vi "Tosca-Configure Multirigs.vi"(2 "Parent VI":refnum<vi>) -> (8 "Canceled?":bool)   [LabVIEW 2020]
uses:
  epl-vi-lib/Utility VIs/Buttons/KCheckmarkBoolean 2.ctl
  epl-vi-lib/Utility VIs/Controls/KTable/KTable.xctl
panel:
  in  "KTable":u16(xcontrol)
  in  "Apply to all":T1
  in  "Edit defaults":bool
  in  "Cancel":bool
  in  "OK":bool
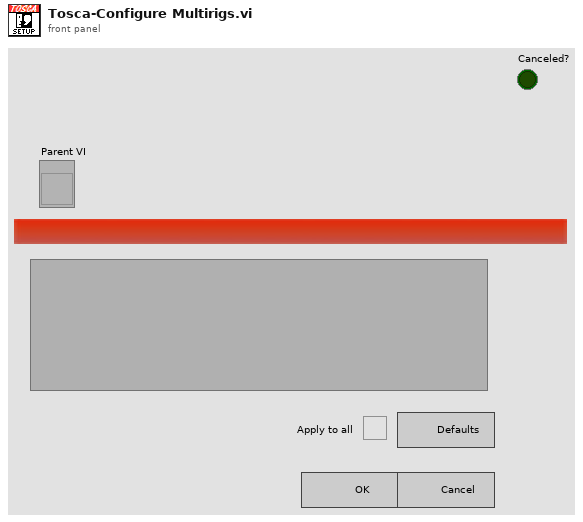
[diagram p1: front panel]
types:
  T1 = typedef "KCheckmarkBoolean 2.ctl" = bool
  T2 = cluster{"Name":string, "Audio":string, "Digital":string, "Video":string}[]
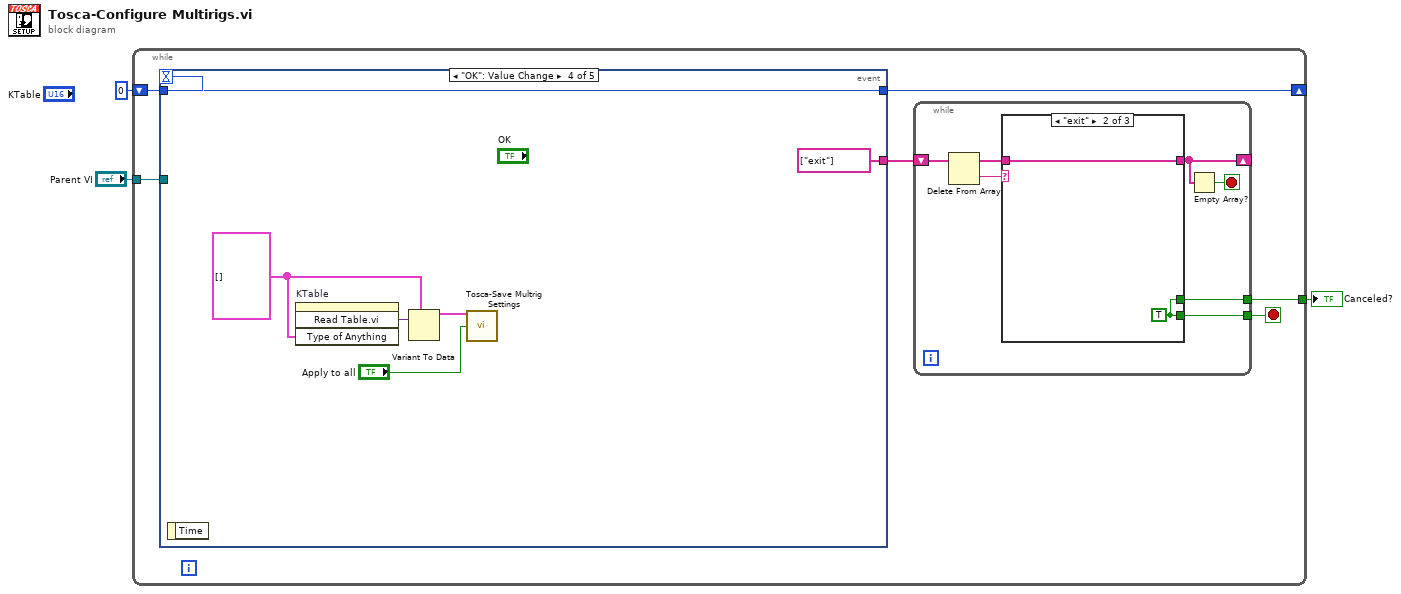
[diagram p0: block diagram]
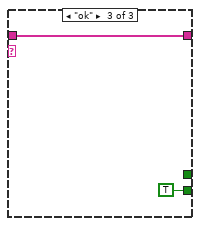
[diagram p3: hidden frame]
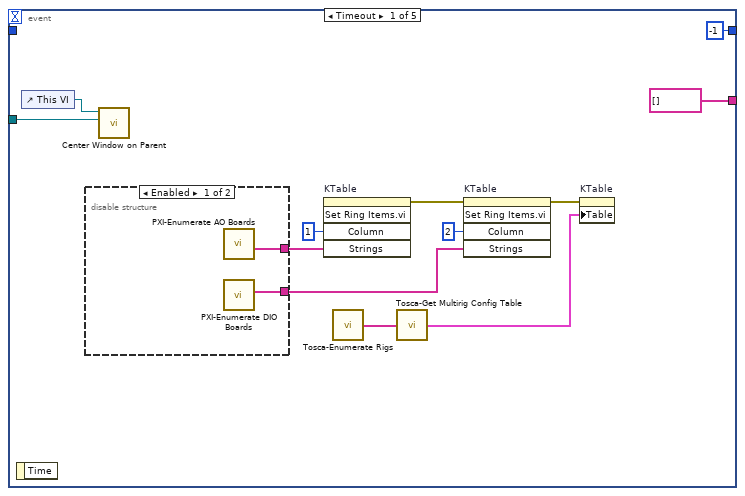
[diagram p4: hidden frame]
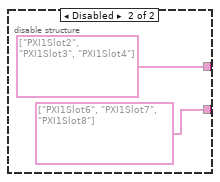
[diagram p5: hidden frame]
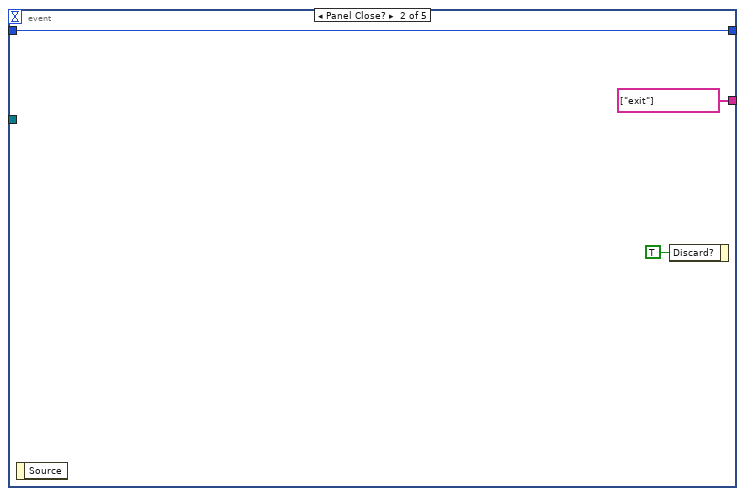
[diagram p6: hidden frame]
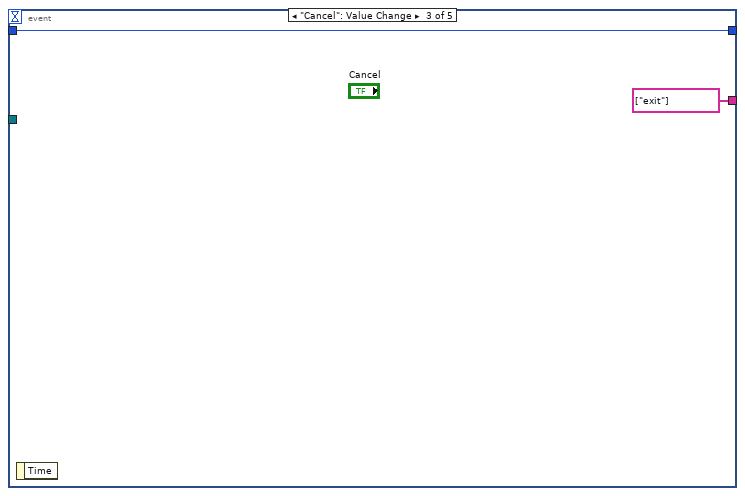
[diagram p7: hidden frame]
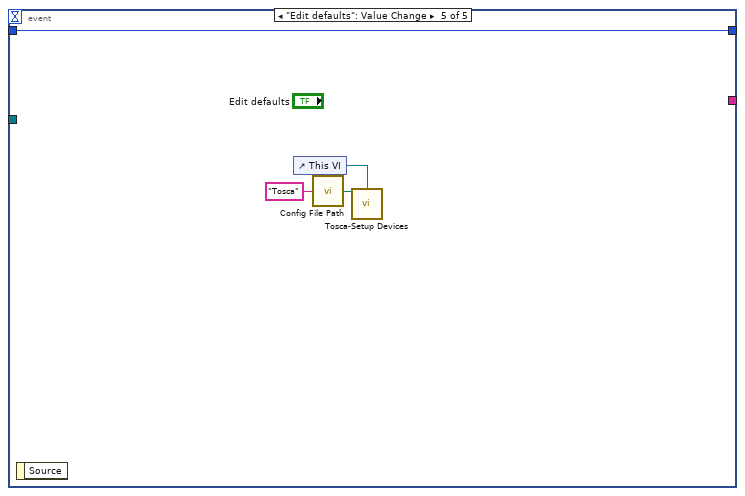
[diagram p8: hidden frame]
diagram:
  n1 = while {
    shift-right: [w9] -> _
    shift-left: 0 -> [w8]
    tunnel: [w5] -> w2
    tunnel: "Parent VI" -> [w4]
    stop <- w6 stop-if-true
    n2 = event shown="[3] \"OK\": Value Change" {
      selector: _ -> [_ _ _ _ _]
      dyn-events: _ -> [_ _ _ _ _]
      timeout: w8 -> [_ _ _ _ _]
      tunnel: [-1 w40 w42 w48 w52] -> w9
      tunnel: w8 -> [_ w40 w42 w48 w52]
      tunnel: [string[] [] string[] ["exit"] string[] ["exit"] string[] ["exit"] _] -> w7
      tunnel: w4 -> [w30 _ _ _ _]
      event Timeout {
        n3 = event-data() -> ()  [unwired: 1 in, 1 out]
        n4 = control-ref of="This VI"() -> (w31:refnum<vi>)
        n5 = disable-structure shown="Enabled" {
          disable-tunnel: [w34 string[] ["PXI1Slot2", "PXI1Slot3", "PXI1Slot4"]] -> w25
          disable-tunnel: [w35 string[] ["PXI1Slot6", "PXI1Slot7", "PXI1Slot8"]] -> w29
          frame Enabled {
            n6 = call "PXI-Enumerate AO Boards.vi"() -> ("24-bit devices"=w34:tag[])  [unwired: 9 in, 2 out]
            n7 = call "PXI-Enumerate DIO Boards.vi"() -> ("Devices"=w35:tag[])  [unwired: 10 in, 1 out]
          }
          frame Disabled {
          }
        }
        n8 = call "Center Window on Parent.vi"("Parent VI"=w30, "VI in"=w31) -> ()  [unwired: 8 in, 2 out]
        n9 = invoke on="KTable" class="KTable (strict)" method="Set Ring Items.vi"("Column"=1, "Strings"=w25) -> (error out=w27:errorcluster)  [unwired: 3 in, 4 out]
        n10 = call "Tosca-Enumerate Rigs.vi"() -> ("Rigs"=w24:string[])  [unwired: 15 in]
        n11 = call "Tosca-Get Multirig Config Table.vi"("Rigs"=w24) -> ("Table"=w22:T2)  [unwired: 14 in]
        n12 = invoke on="KTable" class="KTable (strict)" method="Set Ring Items.vi"(error in=w27, "Column"=2, "Strings"=w29) -> (error out=w23:errorcluster)  [unwired: 2 in, 4 out]
        n13 = property on="KTable" class="KTable (strict)"(error in=w23, "Table"=w22) -> ()  [unwired: 1 in, 2 out]
      }
      event Panel Close? {
        n14 = event-data() -> ()  [unwired: 1 in, 1 out]
        n15 = event-data("Discard?"=TRUE) -> ()  [unwired: 1 in, 1 out]
      }
      event "Cancel": Value Change {
        n16 = event-data() -> ()  [unwired: 1 in, 1 out]
      }
      event "OK": Value Change {
        w46 = cluster{string, string, string, string}[] []
        n17 = event-data() -> ()  [unwired: 1 in, 1 out]
        n18 = invoke on="KTable" class="KTable (strict)" method="Read Table.vi"("Type of Anything"=w46) -> ("Read Table.vi"=w45:variant)  [unwired: 3 in, 3 out]
        n19 = Variant To Data(type=w46, Variant=w45) -> (data=w44:cluster{string, string, string, string}[])  [unwired: 1 in, 1 out]
        n20 = call "Tosca-Save Multrig Settings.vi"("Table"=w44, "Apply defaults"="Apply to all") -> ()  [unwired: 14 in]
      }
      event "Edit defaults": Value Change {
        n21 = event-data() -> ()  [unwired: 1 in, 1 out]
        n22 = control-ref of="This VI"() -> (w50:refnum<vi>)
        n23 = call "Config File Path.vi"("AppName"="Tosca") -> ("Default config file name"=w49:path)
        n24 = call "Tosca-Setup Devices.vi"("Configuration file"=w49, "Parent VI"=w50) -> ()  [unwired: 13 in, 1 out]
      }
    }
    n25 = while {
      shift-right: [w13] -> _
      shift-left: w7 -> [w16]
      tunnel: [w11] -> w6
      tunnel: [w10] -> w5
      stop <- w12 stop-if-true
      n26 = Delete From Array(array=w16) -> (deleted portion=w14:string, array with subset deleted=w15:string[])  [unwired: 2 in]
      n27 = case shown="\"exit\"" w14 {
        tunnel: w15 -> [w17 w19 w21]
        tunnel: [w17 w19 w21] -> w13
        tunnel: [_ w18 TRUE] -> w11
        tunnel: [_ w18 _] -> w10
        frame "", Default {
        }
        frame "exit" {
          w18 = TRUE
        }
        frame "ok" {
        }
      }
      n28 = Empty Array?(array=w13) -> (empty?=w12:bool)
    }
  }
  "Canceled?" <- w2
